vi "Periodic Tasks.vi"(8 "error in":errorcluster) -> ()   [LabVIEW 2016]
doc: "This VI runs in parallel to other tasks. It can contain as many user-defined periodic loops as you need. These can carry out PID or other sorts of timed response."
uses:
  <vilib>/Rock Robotics/WPI/Relay/WPI_RelayValue.ctl
  <vilib>/Rock Robotics/WPI/Utilities/WPI_GetSetVariantRefNum.vi
  AutoaimVar.vi
  Robot Global Data.vi
  <vilib>/Rock Robotics/Network Tables/NT Write Number.vi
  Global Current Values.vi
  <vilib>/Rock Robotics/SystemInterfaces/Utilities/FPGA_UtilitiesRead LocalTime.vi
panel:
  out "Last Autoaim Epsilon":bool
  out "Waveform Graph":dbl[](graph)
  out "Waveform Graph 2":dbl[](graph)
  out "Current Pivot Speed":dbl=0.35
  out "Right Boundary":dbl=-357.80213110000045
  out "Left Boundary":dbl=-387.80213110000045
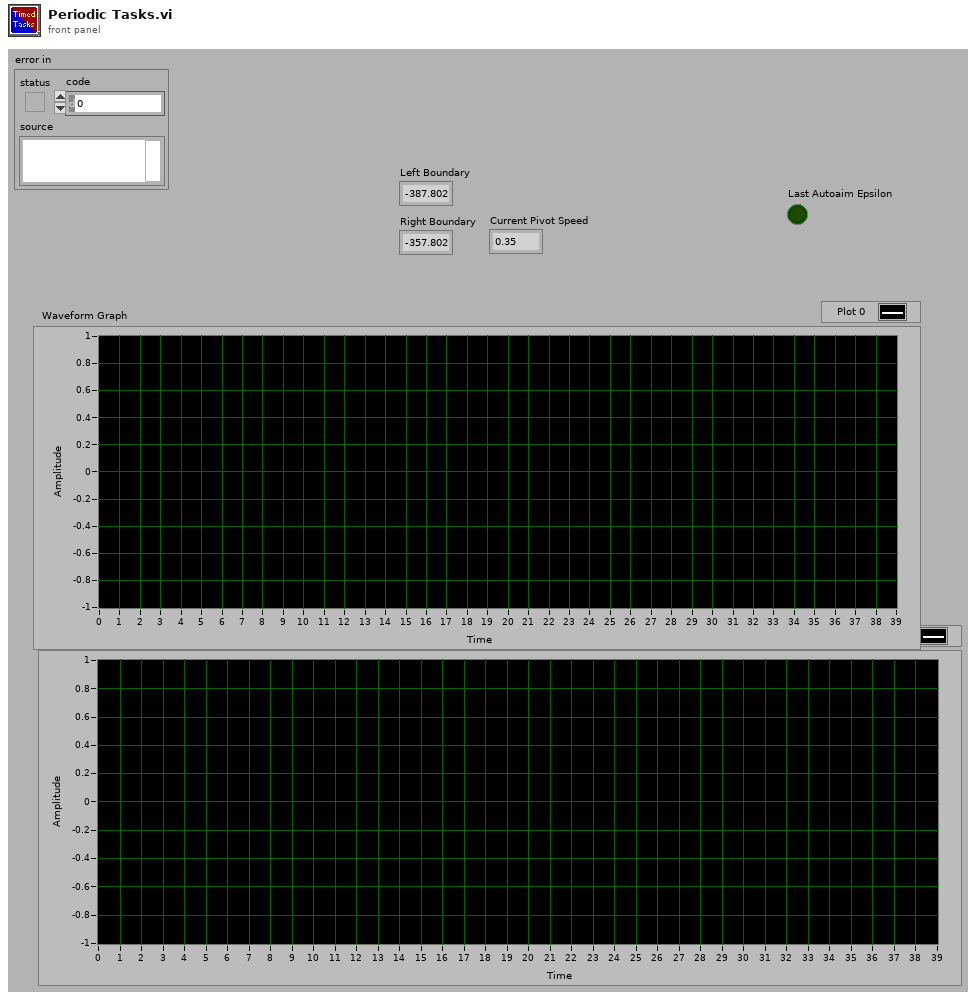
[diagram p1: front panel]
types:
  T1 = cluster{"Yaw":dbl, "Roll":dbl, "Pitch":dbl, "Heading":dbl, "Fused Heading":dbl}
  T2 = typedef "WPI_RobotDriveDevRef.ctl" = cluster{"DevStatus":errorcluster, "Motors[]":T3[], "Square Inputs":bool, "Max Output":dbl}
  T3 = typedef "WPI_MotorControlDeviceRef.ctl" = cluster{"DeviceStatus":errorcluster, "Type":T4, "PWM":cluster{"PWM Channel":T5, "DeadBand":T6}, "CAN":cluster{"Device Number":u8, "SetOutput VI Ref":variant, "GetOutput VI Ref":variant, "Enable VI Ref":variant, "Disable VI Ref":variant, "Data":variant}, "Invert":bool}
  T4 = typedef "WPI_MotorControlType.ctl" = enum16{"PWM", "CAN"}
  T5 = typedef "FPGA_DIOPWMChannel.ctl" = enum8{"PWM 0", "PWM 1", "PWM 2", "PWM 3", "PWM 4", "PWM 5", "PWM 6", "PWM 7", "PWM 8", "PWM 9", "PWM MXP 0", "PWM MXP 1", "PWM MXP 2", "PWM MXP 3", "PWM MXP 4", "PWM MXP 5", "PWM MXP 6", "PWM MXP 7", "PWM MXP 8", "PWM MXP 9", "Invalid"}
  T6 = typedef "WPI_PWMDeadband.ctl" = cluster{"Name":string, "maxPositivePwm":i32, "minPositivePwm":i32, "centerPwm":i32, "maxNegativePwm":i32, "minNegativePwm":i32, "angularRange":u16}
  T7 = typedef "WPI_RelayValue.ctl" = enum16{"Off", "On", "Forward", "Reverse"}
  T8 = typedef "WPI_RelayDevRef.ctl" = cluster{"DevStatus":errorcluster, "Relay Channel":T9, "Relay Direction":T10}
  T9 = typedef "FPGA_DIORelayChannel.ctl" = enum8{"Relay 0", "Relay 1", "Relay 2", "Relay 3", "Invalid"}
  T10 = typedef "WPI_RelayDirection.ctl" = enum16{"Both directions", "Forward only", "Reverse only"}
  T11 = typedef "WPI_GyroDevRef.ctl" = cluster{"DevStatus":errorcluster, "Analog Channel":T12, "Offset":dbl, "Gain (VoltsPerDegree/Second)":dbl, "Gyro Type":enum16{"Analog", "XRS450"}, "Handle":i32, "SPI Bus":T13, "Device Found":bool, "Sample Rate":dbl, "Calibrate On Open":bool}
  T12 = typedef "FPGA_AIChannel.ctl" = enum8{"AI 0", "AI 1", "AI 2", "AI 3", "AI MXP 0", "AI MXP 1", "AI MXP 2", "AI MXP 3", "Invalid"}
  T13 = typedef "spi_bus.ctl" = enum16{"SPI On-Board, CS0", "SPI On-Board, CS1", "SPI On-Board, CS2", "SPI On-Board, CS3", "SPI MXP", "Invalid"}
  T14 = cluster{"Default Value":dbl, "Default Value":dbl}
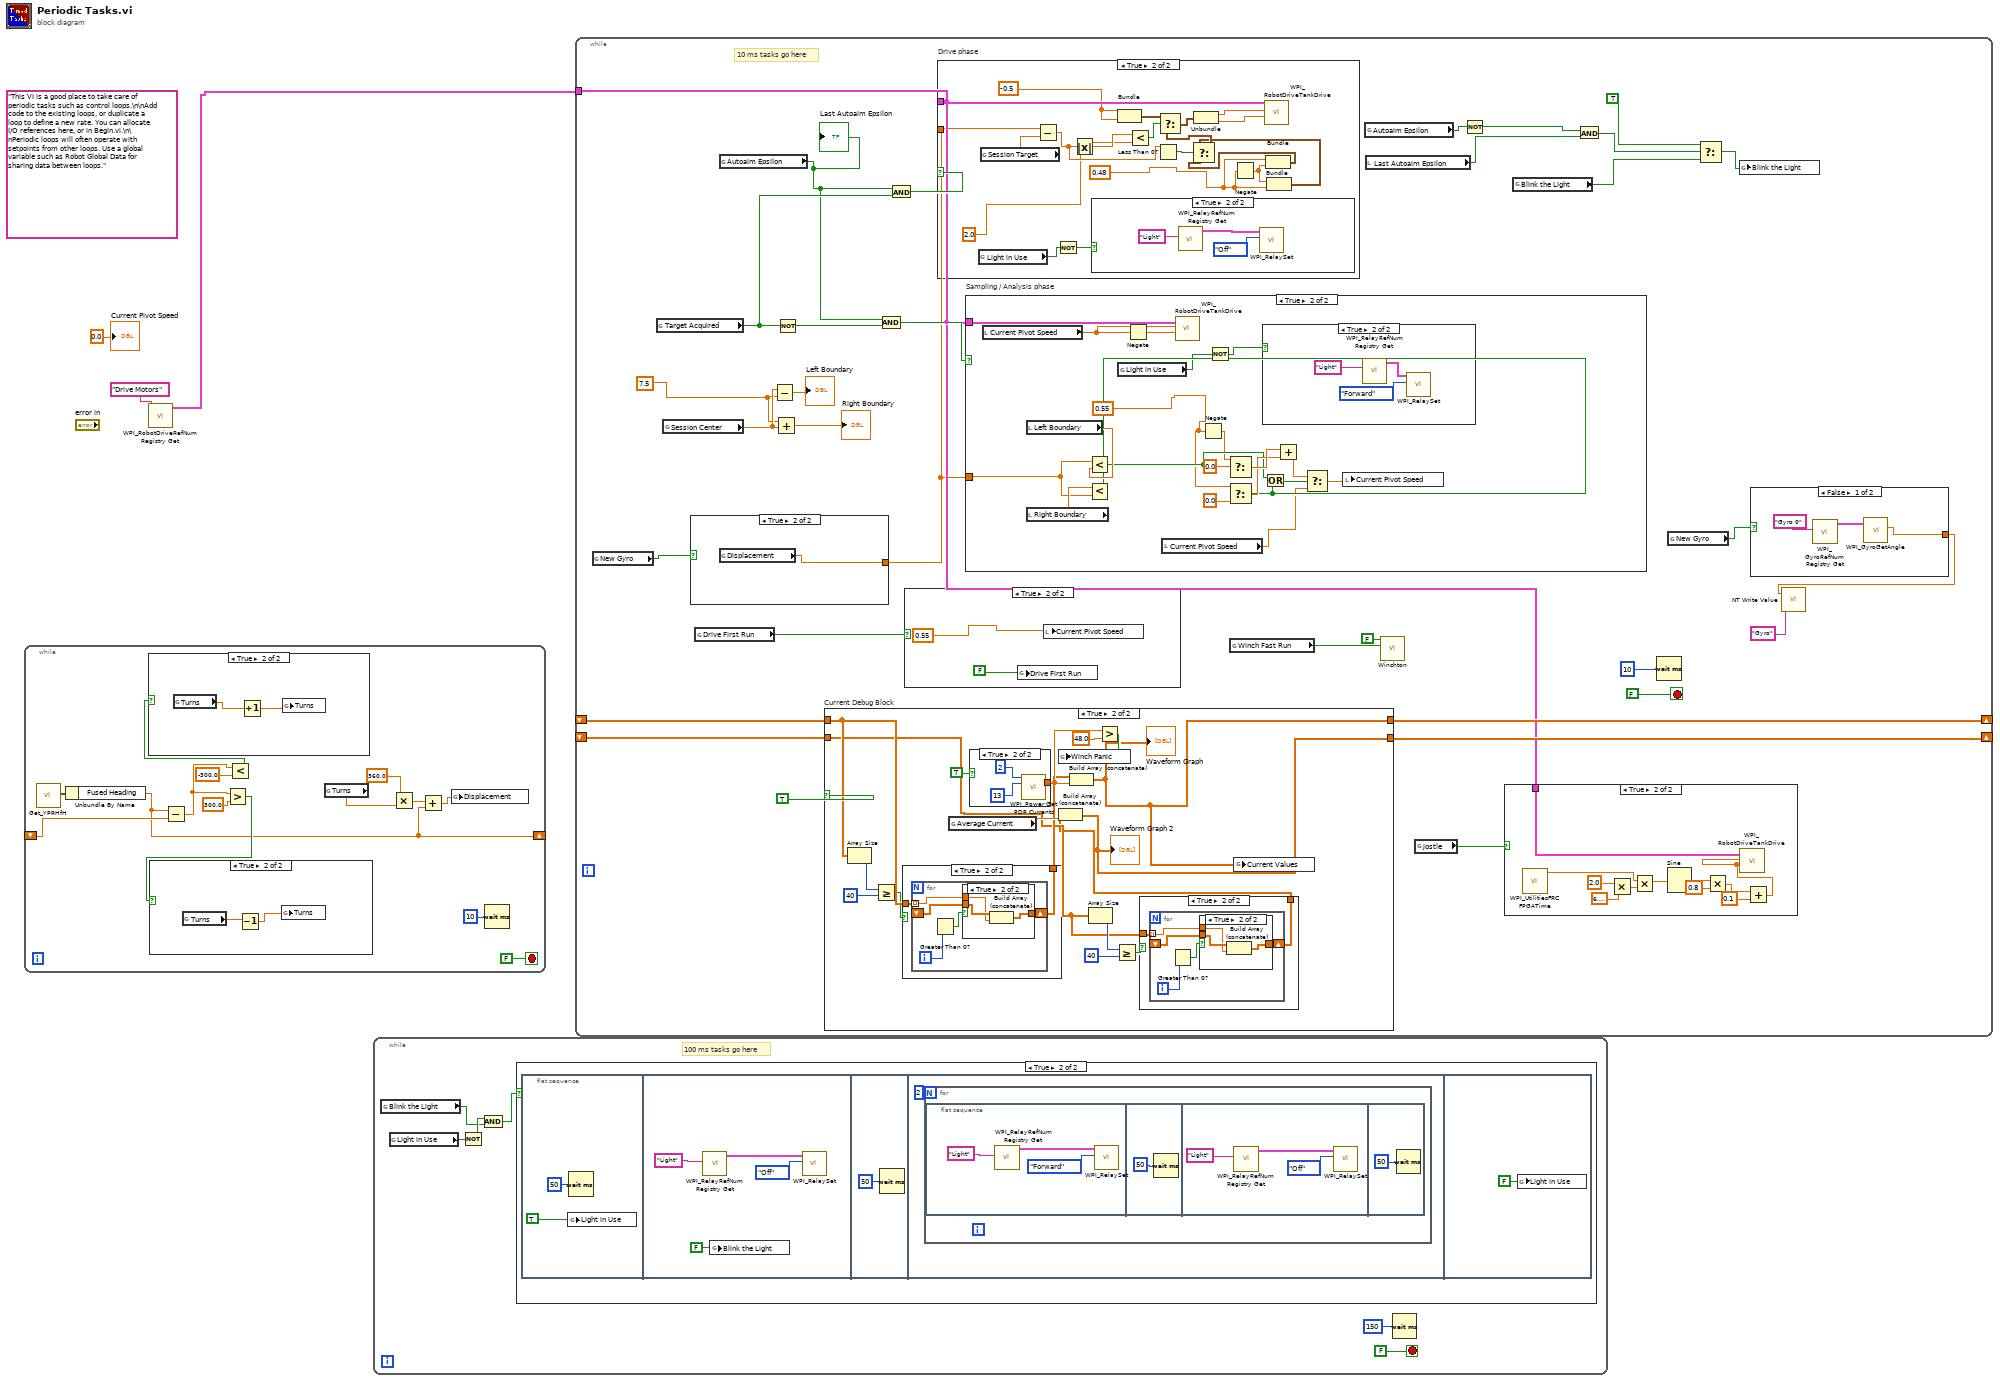
[diagram p0: block diagram]
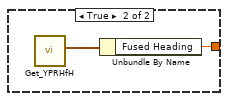
[diagram p5: hidden frame]
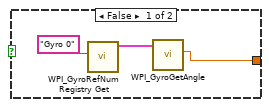
[diagram p6: hidden frame]
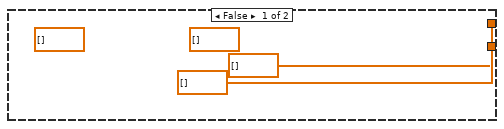
[diagram p8: hidden frame]
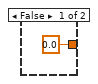
[diagram p9: hidden frame]
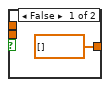
[diagram p11: hidden frame]
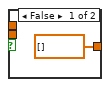
[diagram p13: hidden frame]
diagram:
  (unwired) "This VI is a good place to take care of periodic tasks such as control loops.\n\nAdd code to the existing loops, or duplicate a loop to define a new rate. You can allocate I/O references here, or in Begin.vi.\n\nPeriodic loops will often operate with setpoints from other loops. Use a global variable such as Robot Global Data for sharing data between loops."
  n1 = while {
    shift-right: [w9] -> _
    shift-left: _ -> [w15]
    stop <- FALSE stop-if-true
    n2 = call <vilib>:"Get_YPRHfH.vi"() -> ("YRPHfH"=w17:T1)  [unwired: 11 in]
    n3 = Unbundle By Name(w17) -> ("Fused Heading"=w9:dbl)
    n4 = Subtract(x=w9, y=w15) -> (x-y=w5:dbl)
    n5 = Greater?(x=w5, y=300.0 ("x")) -> (0:w13:bool)
    n6 = case shown="True" w13 {
      frame False {
      }
      frame True {
        n7 = global read "Robot Global Data.vi" "Turns"() -> (w18:dbl)
        n8 = Decrement(x=w18) -> (x-1=w19:dbl)
        n9 = global write "Robot Global Data.vi" "Turns"(w19) -> ()
      }
    }
    n10 = Less?(x=w5, y=-300.0) -> (x < y?=w14:bool)
    n11 = case shown="True" w14 {
      frame False {
      }
      frame True {
        n12 = global read "Robot Global Data.vi" "Turns"() -> (w20:dbl)
        n13 = Increment(x=w20) -> (x+1=w21:dbl)
        n14 = global write "Robot Global Data.vi" "Turns"(w21) -> ()
      }
    }
    n15 = global read "Robot Global Data.vi" "Turns"() -> (w11:dbl)
    n16 = Multiply(x=360.0, y=w11) -> (x*y=w10:dbl)
    n17 = Add(x=w10, y=w9) -> (x+y=w8:dbl)
    n18 = global write "Robot Global Data.vi" "Displacement"(w8) -> ()
    n19 = Wait (ms)(milliseconds to wait=u32 10) -> ()  [unwired: 1 out]
  }
  n20 = call <vilib>:"WPI_RobotDriveRefNum Registry Get.vi"("refnum name"="Drive Motors") -> ("RobotDriveDevRef"=w2:T2)  [unwired: 1 in, 9 out]
  n21 = while {
    stop <- FALSE stop-if-true
    # "100 ms tasks go here"
    n22 = global read "AutoaimVar.vi" "Blink the Light"() -> (w23:bool)
    n23 = global read "AutoaimVar.vi" "Light in Use"() -> (w25:bool)
    n24 = Not(x=w25) -> (.not. x?=w24:bool)
    n25 = And(x=w24, y=w23) -> (x .and. y?=w22:bool)
    n26 = case shown="True" w22 {
      frame False {
      }
      frame True {
        n27 = flat-sequence {
          frame #0 {
            n28 = global write "AutoaimVar.vi" "Light in Use"(TRUE ("Light in Use")) -> ()
            n29 = Wait (ms)(milliseconds to wait=u32 50) -> ()  [unwired: 1 out]
          }
          frame #1 {
            n30 = call <vilib>:"WPI_RelayRefNum Registry Get.vi"("refnum name"="Light") -> ("RelayDevRef"=w33:T8)  [unwired: 9 in, 1 out]
            n31 = global write "AutoaimVar.vi" "Blink the Light"(FALSE ("Blink the Light")) -> ()
            n32 = call <vilib>:"WPI_RelaySet.vi"("RelayValue"=WPI_RelayValue."Off", "RelayDevRef"=w33) -> ()  [unwired: 8 in, 2 out]
          }
          frame #2 {
            n33 = Wait (ms)(milliseconds to wait=u32 50) -> ()  [unwired: 1 out]
          }
          frame #3 {
            n34 = for {
              N: 2 -> [_]
              n35 = flat-sequence {
                frame #0 {
                  n36 = call <vilib>:"WPI_RelayRefNum Registry Get.vi"("refnum name"="Light") -> ("RelayDevRef"=w38:T8)  [unwired: 9 in, 1 out]
                  n37 = call <vilib>:"WPI_RelaySet.vi"("RelayValue"=WPI_RelayValue."Forward", "RelayDevRef"=w38) -> ()  [unwired: 8 in, 2 out]
                }
                frame #1 {
                  n38 = Wait (ms)(milliseconds to wait=u32 50) -> ()  [unwired: 1 out]
                }
                frame #2 {
                  n39 = call <vilib>:"WPI_RelayRefNum Registry Get.vi"("refnum name"="Light") -> ("RelayDevRef"=w42:T8)  [unwired: 9 in, 1 out]
                  n40 = call <vilib>:"WPI_RelaySet.vi"("RelayValue"=WPI_RelayValue."Off", "RelayDevRef"=w42) -> ()  [unwired: 8 in, 2 out]
                }
                frame #3 {
                  n41 = Wait (ms)(milliseconds to wait=u32 50) -> ()  [unwired: 1 out]
                }
              }
            }
          }
          frame #4 {
            n42 = global write "AutoaimVar.vi" "Light in Use"(FALSE ("Light in Use")) -> ()
          }
        }
      }
    }
    n43 = Wait (ms)(milliseconds to wait=u32 150) -> ()  [unwired: 1 out]
  }
  n44 = while {
    tunnel: w2 -> [w50]
    shift-right: [w65] -> _
    shift-left: _ -> [w64]
    shift-right: [w63] -> _
    shift-left: _ -> [w62]
    stop <- FALSE stop-if-true
    w49 = 7.5 ("x")
    # "10 ms tasks go here"
    n45 = global read "Robot Global Data.vi" "New Gyro"() -> (w47:bool)
    n46 = global read "AutoaimVar.vi" "Target Acquired"() -> (w69:bool)
    n47 = global read "AutoaimVar.vi" "Session Center"() -> (w74:dbl)
    n48 = case shown="True" w47 {
      tunnel: [w83 w86] -> w48
      frame False {
        n49 = call <vilib>:"WPI_GyroRefNum Registry Get.vi"("refnum name"="Gyro 0") -> ("GyroDevRef"=w84:T11)  [unwired: 9 in, 1 out]
        n50 = call <vilib>:"WPI_GyroGetAngle.vi"("GyroDevRef"=w84) -> ("Angle"=w83:dbl)  [unwired: 6 in, 4 out]
      }
      frame True {
        n51 = global read "Robot Global Data.vi" "Displacement"() -> (w86:dbl)
      }
    }
    n52 = global read "AutoaimVar.vi" "Drive First Run"() -> (w70:bool)
    n53 = global read "AutoaimVar.vi" "Autoaim Epsilon"() -> (w60:bool)
    "Last Autoaim Epsilon" <- w60
    n54 = Subtract(x=w74, y=w49) -> (x-y=→"Left Boundary":dbl)
    n55 = Add(x=w49, y=w74) -> (x+y=→"Right Boundary":dbl)
    n56 = Not(x=w69) -> (.not. x?=w68:bool)
    n57 = case "Current Debug Block" shown="True" TRUE {
      tunnel: [dbl[] [] w113] -> w63
      tunnel: w62 -> [_ w102]
      tunnel: [dbl[] [] w111] -> w65
      tunnel: w64 -> [_ w109]
      frame False {
        (unwired) dbl[] []
        (unwired) dbl[] []
      }
      frame True {
        n58 = Array Size(array=w109) -> (size(s)=w107:i32)
        n59 = Greater Or Equal?(x=w107, y=40) -> (x >= y?=w108:bool)
        n60 = case shown="True" w108 {
          tunnel: w109 -> [w133 w135]
          tunnel: [w133 w134] -> w110
          frame False {
          }
          frame True {
            n61 = for {
              tunnel: w135 -> [w136] mode=indexing
              shift-right: [w137] -> w134
              shift-left: _ -> [w138]
              i -> [w140]
              n62 = Greater Than 0?(x=w140) -> (x > 0?=w139:bool)
              n63 = case shown="True" w139 {
                tunnel: w138 -> [_ w144]
                tunnel: [dbl[] [] w143] -> w137
                tunnel: w136 -> [_ w142]
                frame False {
                }
                frame True {
                  n64 = Build Array (concatenate)(w144, w142) -> (w143:dbl[])
                }
              }
            }
          }
        }
        n65 = global read "Global Current Values.vi" "Average Current"() -> (w112:dbl)
        n66 = case shown="True" TRUE {
          tunnel: [0.0 ("current (A)") w118] -> w116
          frame False {
          }
          frame True {
            n67 = call <vilib>:"WPI_Power Get PDP Currents.vi"("Power Distribution Panel (0)"=u8 2, "PDP Channel"=13) -> ("current (A)"=w118:dbl)  [unwired: 11 in, 2 out]
          }
        }
        n68 = Build Array (concatenate)(w110, w116) -> (w111:dbl[])
        "Waveform Graph" <- w111
        n69 = Array Size(array=w102) -> (size(s)=w104:i32)
        n70 = Greater?(x=w116, y=48.0) -> (0:w114:bool)
        n71 = global write "AutoaimVar.vi" "Winch Panic"(w114) -> ()
        n72 = Greater Or Equal?(x=w104, y=40) -> (x >= y?=w105:bool)
        n73 = case shown="True" w105 {
          tunnel: w102 -> [w121 w123]
          tunnel: [w121 w122] -> w101
          frame False {
          }
          frame True {
            n74 = for {
              tunnel: w123 -> [w124] mode=indexing
              shift-right: [w125] -> w122
              shift-left: _ -> [w126]
              i -> [w128]
              n75 = Greater Than 0?(x=w128) -> (x > 0?=w127:bool)
              n76 = case shown="True" w127 {
                tunnel: w126 -> [_ w132]
                tunnel: [dbl[] [] w131] -> w125
                tunnel: w124 -> [_ w130]
                frame False {
                }
                frame True {
                  n77 = Build Array (concatenate)(w132, w130) -> (w131:dbl[])
                }
              }
            }
          }
        }
        n78 = Build Array (concatenate)(w101, w112) -> (w113:dbl[])
        "Waveform Graph 2" <- w113
        n79 = global write "Global Current Values.vi" "Current Values"(w111) -> ()
      }
    }
    n80 = And(x=w60, y=w68) -> (x .and. y?=w73:bool)
    n81 = And(x=w60, y=w69) -> (x .and. y?=w75:bool)
    n82 = case shown="True" w70 {
      frame False {
      }
      frame True {
        n83 = global write "AutoaimVar.vi" "Drive First Run"(FALSE ("Drive First Run")) -> ()
        n84 = local write "Current Pivot Speed"(0.55 ("Default Value")) -> ()
      }
    }
    n85 = case "Drive phase" shown="True" w75 {
      tunnel: w50 -> [_ w189]
      tunnel: w48 -> [_ w188]
      frame False {
      }
      frame True {
        w171 = -0.5 ("Default Value")
        w170 = 0.48 ("Default Value")
        n86 = global read "AutoaimVar.vi" "Light in Use"() -> (w173:bool)
        n87 = global read "AutoaimVar.vi" "Session Target"() -> (w187:dbl)
        n88 = Subtract(x=w188, y=w187) -> (x-y=w179:dbl)
        n89 = Not(x=w173) -> (.not. x?=w174:bool)
        n90 = Absolute Value(x=w179) -> (abs(x)=w186:dbl)
        n91 = case shown="True" w174 {
          frame False {
          }
          frame True {
            n92 = call <vilib>:"WPI_RelayRefNum Registry Get.vi"("refnum name"="Light") -> ("RelayDevRef"=w192:T8)  [unwired: 9 in, 1 out]
            n93 = call <vilib>:"WPI_RelaySet.vi"("RelayValue"=WPI_RelayValue."Off", "RelayDevRef"=w192) -> ()  [unwired: 8 in, 2 out]
          }
        }
        n94 = Bundle("Default Value"=w171, "Default Value"=w171) -> (w184:T14)  [unwired: 1 in]
        n95 = Less?(x=w186, y=2.0 ("Default Value")) -> (x < y?=w185:bool)
        n96 = Less Than 0?(x=w179) -> (x < 0?=w178:bool)
        n97 = Negate(x=w170) -> (-x=w180:dbl)
        n98 = Bundle("Default Value"=w170, w180) -> (w176:cluster{"Default Value":dbl, dbl})  [unwired: 1 in]
        n99 = Bundle(w180, "Default Value"=w170) -> (w175:cluster{dbl, "Default Value":dbl})  [unwired: 1 in]
        n100 = Select(t=w175, s=w178, f=w176) -> (s? t:f=w177:T14)
        n101 = Select(t=w184, s=w185, f=w177) -> (s? t:f=w183:T14)
        n102 = Unbundle(w183) -> ("Default Value"=w182:dbl, "Default Value"=w181:dbl)
        n103 = call <vilib>:"WPI_RobotDriveTankDrive.vi"("Right axis value"=w181, "Left axis value"=w182, "RobotDriveDevRef"=w189) -> ()  [unwired: 6 in, 3 out]
      }
    }
    n104 = case "Sampling / Analysis phase" shown="True" w73 {
      tunnel: w50 -> [_ w166]
      tunnel: w48 -> [_ w152]
      frame False {
      }
      frame True {
        w147 = 0.55 ("Default Value")
        n105 = local read "Current Pivot Speed"() -> (w153:dbl)
        n106 = local read "Left Boundary"() -> (w165:dbl)
        n107 = local read "Right Boundary"() -> (w164:dbl)
        n108 = Less?(x=w152, y=w165) -> (x < y?=w156:bool)
        n109 = Less?(x=w164, y=w152) -> (x < y?=w157:bool)
        n110 = global read "AutoaimVar.vi" "Light in Use"() -> (w149:bool)
        n111 = Negate(x=w153) -> (-x=w154:dbl)
        n112 = local read "Current Pivot Speed"() -> (w151:dbl)
        n113 = call <vilib>:"WPI_RobotDriveTankDrive.vi"("Right axis value"=w154, "Left axis value"=w153, "RobotDriveDevRef"=w166) -> ()  [unwired: 6 in, 3 out]
        n114 = Negate(x=w147) -> (-x=w150:dbl)
        n115 = Not(x=w149) -> (.not. x?=w148:bool)
        n116 = Select(t=w150, s=w156, f=0.0) -> (s? t:f=w161:dbl)
        n117 = Select(t=w147, s=w157, f=0.0) -> (s? t:f=w160:dbl)
        n118 = case shown="True" w148 {
          frame False {
          }
          frame True {
            n119 = call <vilib>:"WPI_RelayRefNum Registry Get.vi"("refnum name"="Light") -> ("RelayDevRef"=w169:T8)  [unwired: 9 in, 1 out]
            n120 = call <vilib>:"WPI_RelaySet.vi"("RelayValue"=WPI_RelayValue."Forward", "RelayDevRef"=w169) -> ()  [unwired: 8 in, 2 out]
          }
        }
        n121 = Or(x=w156, y=w157) -> (x .or. y?=w158:bool)
        n122 = Add(x=w161, y=w160) -> (x+y=w159:dbl)
        n123 = Select(t=w159, s=w158, f=w151) -> (s? t:f=w155:dbl)
        n124 = local write "Current Pivot Speed"(w155) -> ()
      }
    }
    n125 = global read "AutoaimVar.vi" "Winch Fast Run"() -> (w67:bool)
    n126 = global read "AutoaimVar.vi" "Autoaim Epsilon"() -> (w59:bool)
    n127 = local read "Last Autoaim Epsilon"() -> (w57:bool)
    n128 = call "Winchton.vi"("Auto Drive Button"=w67, "Joystickbutton"=FALSE) -> ()  [unwired: 10 in]
    n129 = global read "AutoaimVar.vi" "jostle"() -> (w51:bool)
    n130 = Not(x=w59) -> (.not. x?=w58:bool)
    n131 = case shown="True" w51 {
      tunnel: w50 -> [_ w97]
      frame False {
      }
      frame True {
        n132 = call <vilib>:"WPI_UtilitiesFRC FPGATime.vi"() -> ("FPGA Time"=w93:dbl)  [unwired: 10 in, 1 out]
        n133 = Multiply(x=2.0, y=6.283185307179586) -> (x*y=w94:dbl)
        n134 = Multiply(x=w93, y=w94) -> (x*y=w92:dbl)
        n135 = Sine(x=w92) -> (sin(x)=w91:dbl)
        n136 = Multiply(x=w91, y=0.8) -> (x*y=w89:dbl)
        n137 = Add(x=w89, y=0.1) -> (x+y=w87:dbl)
        n138 = call <vilib>:"WPI_RobotDriveTankDrive.vi"("Right axis value"=w87, "Left axis value"=w87, "RobotDriveDevRef"=w97) -> ()  [unwired: 6 in, 3 out]
      }
    }
    n139 = global read "AutoaimVar.vi" "Blink the Light"() -> (w55:bool)
    n140 = And(x=w58, y=w57) -> (x .and. y?=w56:bool)
    n141 = Wait (ms)(milliseconds to wait=u32 10) -> ()  [unwired: 1 out]
    n142 = global read "Robot Global Data.vi" "New Gyro"() -> (w46:bool)
    n143 = Select(t=TRUE, s=w56, f=w55) -> (s? t:f=w54:bool)
    n144 = global write "AutoaimVar.vi" "Blink the Light"(w54) -> ()
    n145 = case shown="False" w46 {
      tunnel: [w78 w81] -> w45
      frame False {
        n146 = call <vilib>:"WPI_GyroRefNum Registry Get.vi"("refnum name"="Gyro 0") -> ("GyroDevRef"=w79:T11)  [unwired: 9 in, 1 out]
        n147 = call <vilib>:"WPI_GyroGetAngle.vi"("GyroDevRef"=w79) -> ("Angle"=w78:dbl)  [unwired: 6 in, 4 out]
      }
      frame True {
        n148 = call <vilib>:"Get_YPRHfH.vi"() -> ("YRPHfH"=w82:T1)  [unwired: 11 in]
        n149 = Unbundle By Name(w82) -> ("Fused Heading"=w81:dbl)
      }
    }
    n150 = call-poly <vilib>:"NT Write Value.vi"("Numeric"=w45, "Name"="Gyro") -> ()  [unwired: 9 in, 1 out]
  }
  "Current Pivot Speed" <- 0.0 ("Current Pivot Speed")
